vi "Launch Async Threads.vi"(7 "thread count":i32=1, 8 "error in (no error)":errorcluster, 10 "Plugin Thread":refnum<class "Plugin Thread.lvclass">, 11 "Plugin in":refnum<class "Plugin.lvclass">) -> (0 "error out":errorcluster, 3 "Plugin out":refnum<class "Plugin.lvclass">)   [LabVIEW 2017, in "DSF Core.lvlib" / "Plugin.lvclass"]
uses:
  Plugin.lvclass
  Transceiver/Plugin Thread.lvclass
  Plugin.lvclass/Plugin.ctl
  Timing/Timing.lvclass/Timing.ctl
  Debug/Debug Flags/Debug Flags.lvclass/Debug Flags.ctl
  Thread Pool/Pool.lvclass/Pool.ctl
  Debug/FIFO Flags/FIFO Flags.lvclass/FIFO Flags.ctl
  Thread Pool/Read FIFO.vi
  Thread Pool/Write FIFO.vi
  Thread Pool/Get FIFO.vi
  Debug/FIFO Flags/Get Infinite Timeouts.vi
  Thread Pool/ID Pool.lvclass
  C:/Git/DSF/Data Sharing Framework/Source/Core/Engine/Classes/Thread Pool/Pool.lvclass
  Thread Pool/Errors.vi
  Thread Pool/Obtain ID Timeout.vi
  Thread Pool/Return ID Timeout.vi
  Thread Parameters/Thread Parameters.lvclass
  Timing/Timing.lvclass
  Debug/Debug Flags/Debug Flags.lvclass
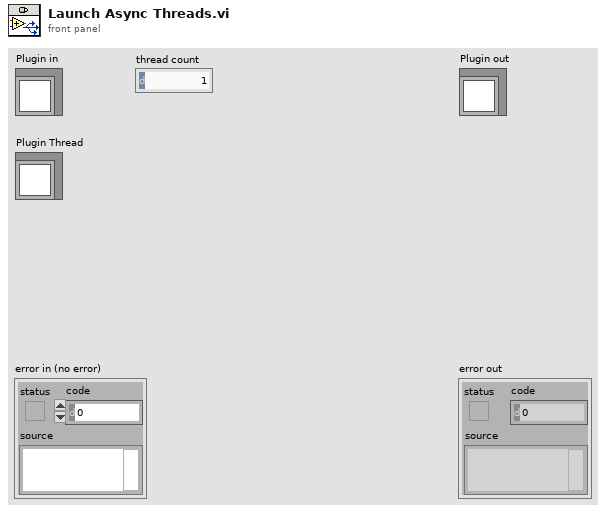
[diagram p1: front panel]
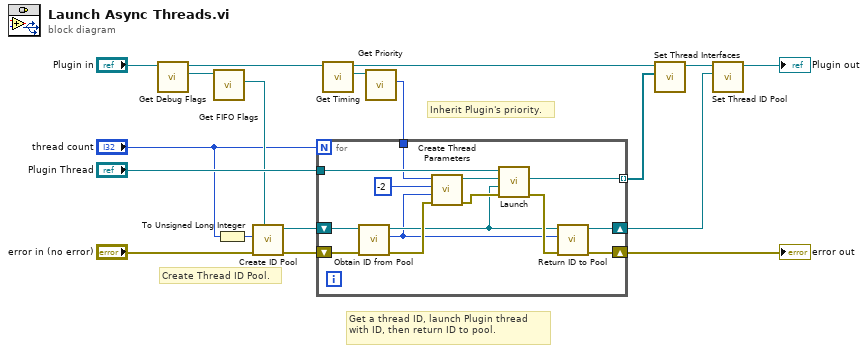
[diagram p0: block diagram]
diagram:
  # "Inherit Plugin's priority."
  # "Get a thread ID, launch Plugin thread with ID, then return ID to pool."
  # "Create Thread ID Pool."
  n1 = call "Get Debug Flags.vi"("Plugin in"="Plugin in") -> ("Debug Flags"=w6:refnum<class "Debug Flags.lvclass">, "Plugin out"=w18:refnum<class "Plugin.lvclass">)  [unwired: 9 in]
  n2 = call "Get FIFO Flags.vi"("Debug Flags in"=w6) -> ("FIFO"=w2:refnum<class "FIFO Flags.lvclass">)  [unwired: 9 in, 1 out]
  n3 = To Unsigned Long Integer(number="thread count") -> (unsigned 32bit integer=w12:u32)
  n4 = call "Create ID Pool.vi"("FIFO Debug Flags"=w2, "error in (no error)"="error in (no error)", "number of IDs"=w12) -> ("error out"=w7:errorcluster, "ID Pool out"=w13:refnum<class "ID Pool.lvclass">)  [unwired: 7 in]
  n5 = call "Get Timing.vi"("Plugin in"=w18) -> ("Timing"=w15:refnum<class "Timing.lvclass">, "Plugin out"=w4:refnum<class "Plugin.lvclass">)  [unwired: 9 in]
  n6 = call "Get Priority.vi"("Timing in"=w15) -> ("Priority"=w14:u64)  [unwired: 9 in, 1 out]
  n7 = for {
    N: "thread count" -> [_]
    shift-right: [w24] -> w17
    shift-left: w7 -> [w21]
    tunnel: w14 -> [w19]
    tunnel: [w25] -> w11 mode=indexing
    shift-right: [w22] -> w8
    shift-left: w13 -> [w23]
    tunnel: "Plugin Thread" -> [w20]
    n8 = call "Obtain ID from Pool.vi"("error in (no error)"=w21, "ID Pool in"=w23) -> ("error out"=w31:errorcluster, "id"=w26:i32, "ID Pool out"=w28:refnum<class "ID Pool.lvclass">)  [unwired: 6 in, 1 out]
    n9 = call "Create Thread Parameters.vi"("error in (no error)"=w31, "id (0)"=w26, "processor (-2)"=-2 ("processor"), "priority (100)"=w19) -> ("error out"=w30:errorcluster, "Thread Parameters"=w27:refnum<class "Thread Parameters.lvclass">)  [unwired: 6 in]
    n10 = call "Launch.vi"("error in (no error)"=w30, "Thread ID Pool"=w28, "Thread Parameters"=w27, "Plugin Thread in"=w20) -> ("error out"=w29:errorcluster, "Interface"=w25:refnum<class "Plugin Interface.lvclass">)  [unwired: 5 in, 1 out]
    n11 = call "Return ID to Pool.vi"("error in (no error)"=w29, "id"=w26, "ID Pool in"=w28) -> ("error out"=w24:errorcluster, "ID Pool out"=w22:refnum<class "ID Pool.lvclass">)  [unwired: 6 in, 1 out]
  }
  "error out" <- w17
  n12 = call "Set Thread Interfaces.vi"("Plugin Interfaces"=w11, "Plugin in"=w4) -> ("Plugin out"=w10:refnum<class "Plugin.lvclass">)  [unwired: 9 in]
  n13 = call "Set Thread ID Pool.vi"("Thread ID Pool"=w8, "Plugin in"=w10) -> ("Plugin out"=→"Plugin out":refnum<class "Plugin.lvclass">)  [unwired: 9 in]
